vi "BonOMM-SAOMM.vi"() -> ()   [LabVIEW 2019] (continued)
                  tunnel: w3763 -> [w3827]
                  tunnel: [w3827] -> w3762
                  tunnel: w3762 -> [w3840]
                  frame #0 {
                    n5058 = Tick Count (ms)() -> (millisecond timer value=w3793:u32)
                  }
                  frame #1 {
                    # "Détecte un déplacement du télescope"
                    # "Détecte un changement de focus"
                    # "Bits du statut du TCS"
                    n5059 = Index Array(array=w3831, index #1=2 ("Index"), index #2=0 ("Index")) -> (element #1=w3812:bool, element #2=w3815:bool)
                    "Mode Est" <- w3812
                    "Focus slew" <- w3815
                    n5060 = Index Array(array=w3833, index=4 ("Index")) -> (element=w3822:bool)
                    "Target OutofRange" <- w3822
                    n5061 = Index Array(array=w3833, index=0 ("Index")) -> (element=w3804:bool)
                    n5062 = Index Array(array=w3834, index=2 ("Index")) -> (element=→"Tracking":bool)
                    n5063 = Index Array(array=w3834, index=3 ("Index")) -> (element=→"Slew enabled":bool)
                    n5064 = Index Array(array=w3834, index=4 ("indice")) -> (element=w3820:bool)
                    n5065 = Index Array(array=w3834, index=5 ("Index")) -> (element=w3821:bool)
                    "Approaching limit" <- w3821
                    n5066 = Index Array(array=w3834, index=7 ("Index")) -> (element=w3806:bool)
                    "Slewing" <- w3806
                    n5067 = Not Equal?(x=w3804, y=w3828) -> (x != y?=w3805:bool)
                    n5068 = property on="Mode Inversé" class="Bool (strict)"("Visible"=w3812, "Blinking"=w3812) -> ()  [unwired: 2 in, 2 out]
                    n5069 = property on="Target OutofRange" class="Bool (strict)"("Visible"=w3822, "Blinking"=w3822) -> ()  [unwired: 2 in, 2 out]
                    n5070 = local write "Coupole-Tél"(w3820) -> ()
                    n5071 = Not Equal?(x=w3815, y=w3829) -> (x != y?=w3814:bool)
                    n5072 = property on="Approaching limit" class="Bool (strict)"("Visible"=w3821, "Blinking"=w3821) -> ()  [unwired: 2 in, 2 out]
                    n5073 = case shown="Vrai" w3805 {
                      tunnel: w3804 -> [_ w3836]
                      frame False {
                      }
                      frame True {
                        n5074 = property on="Setting" class="Bool (strict)"("Val(Sgnl)"=w3836) -> ()  [unwired: 2 in, 2 out]
                      }
                    }
                    n5075 = case shown="Vrai" w3814 {
                      tunnel: w3815 -> [_ w3837]
                      frame False {
                      }
                      frame True {
                        n5076 = property on="Focus slew" class="Bool (strict)"("Value (Signaling)"=w3837) -> ()  [unwired: 2 in, 2 out]
                      }
                    }
                    n5077 = Not Equal?(x=w3806, y=w3830) -> (x != y?=w3807:bool)
                    n5078 = property on="Slewing" class="Bool (strict)"("Blinking"=w3806) -> ()  [unwired: 2 in, 2 out]
                    n5079 = And(x=w3804, y=w3805) -> (x .and. y?=w3808:bool)
                    n5080 = And(x=w3806, y=w3807) -> (x .and. y?=w3809:bool)
                    n5081 = local read "Servo"() -> (w3801:bool)
                    n5082 = Or(x=w3808, y=w3809) -> (x .or. y?=w3802:bool)
                    n5083 = And(x=w3802, y=w3801) -> (x .and. y?=w3803:bool)
                    n5084 = case shown="Vrai" w3803 {
                      selector: w3803 -> [_ w3835]
                      frame False {
                      }
                      frame True {
                        n5085 = property on="StopServo" class="Bool (strict)"("Val(Sgnl)"=w3835) -> ()  [unwired: 2 in, 2 out]
                      }
                    }
                    n5086 = case shown="Vrai" w3807 {
                      tunnel: w3806 -> [_ w3838]
                      frame False {
                      }
                      frame True {
                        n5087 = property on="Slewing" class="Bool (strict)"("Value (Signaling)"=w3838) -> ()  [unwired: 2 in, 2 out]
                      }
                    }
                    "STATH" <- w3833
                    "STATLH" <- w3832
                    "STATEX" <- w3831
                    "STATL" <- w3834
                  }
                  frame #2 {
                    n5088 = Tick Count (ms)() -> (millisecond timer value=w3841:u32)
                    n5089 = Subtract(x=w3841, y=w3840) -> (x-y=→"TCS #26 (sort)":u32)
                  }
                }
              }
              frame #4 {
                n5090 = Tick Count (ms)() -> (millisecond timer value=w3844:u32)
                n5091 = Subtract(x=w3844, y=w3843) -> (x-y=→"TCS #26":u32)
              }
              frame #5 {
                # "Malheureusement, semble causé un problème \nquand on tente de reconnecté les tables ...\nChecher à comprendre c'Est avoir mal à la tête\nprobablement un VI non-réentrant partager entre\nle query de TCS et le query des tables ..."
                # "Patch pour l'angle (2013/06/22)\nÀ mettre au propre ... attention,\ncela à beaucoup d'impact sur beaucou\nde sous-routine ... (voir tout ce qui re-\nçoit l'angle à un moment)"
                # "À remettre dans un mode correct"
                n5092 = local read "TCSMute"() -> (w3845:bool)
                n5093 = local read "TCS VRN"() -> (w3858:refnum<visa-resource-name>)
                n5094 = control-ref of="TCS actif"() -> (w3856:refnum<vi>)
                n5095 = local read "dflt-EQX"() -> (w3855:dbl)
                n5096 = case shown="Faux" w3845 {
                  tunnel: [w3896 w3897] -> w3879
                  tunnel: [w3895 w3897] -> w3878
                  tunnel: [w3894 w3897] -> w3877
                  tunnel: [w3893 w3897] -> w3876
                  tunnel: [w3892 ""] -> w3875
                  tunnel: [w3891 w3897] -> w3868
                  tunnel: [w3890 w3897] -> w3867
                  tunnel: [w3889 w3897] -> w3866
                  tunnel: [w3888 w3897] -> w3865
                  tunnel: [w3887 errorcluster {"status"=FALSE, "code"=0, "source"=""} ("Error OUT")] -> w3864
                  tunnel: [w3886 w3900] -> w3859
                  tunnel: w3858 -> [w3885 w3900]
                  tunnel: w3856 -> [w3884 _]
                  tunnel: w3855 -> [w3883 _]
                  tunnel: [w3882 w3897] -> w3853
                  tunnel: [w3881 w3897] -> w3852
                  tunnel: [w3880 w3897] -> w3848
                  frame False {
                    n5097 = call "EXCOM-25-EQ.vi"("VISA resource name"=w3885, "Bool Refnum"=w3884, "Display Equinox"=w3883) -> ("HA"=w3893:dbl, "Q String"=w3892:string, "RA"=w3881:dbl, "Rotateur"=w3880:dbl, "DEC"=w3882:dbl, "Dome"=w3896:dbl, "Epoque"=w3891:dbl, "Focus"=w3895:dbl, "VISA resource name dup"=w3886:refnum<visa-resource-name>, "Masse d'air"=w3894:dbl, "Temps Sidéral"=w3890:dbl, "Temps Universel"=w3889:dbl, "Année"=w3888:dbl, "Error OUT"=w3887:errorcluster)  [unwired: 2 in, 1 out]
                  }
                  frame True {
                    w3897 = 0.0
                  }
                }
                "Q String" <- w3875
                "RA Tel" <- w3852
                "DEC Tel" <- w3853
                "Angle Hor." <- w3876
                "Epoch Tel" <- w3868
                "Air Mass" <- w3877
                "LST" <- w3867
                "UTC" <- w3866
                "AnnéeRL" <- w3865
                "Foyer" <- w3878
                "Coupole" <- w3879
                n5098 = call-poly "PolyCommError.vi"("VISA IN"=w3859, "error IN"=w3864) -> ("VISA OUT"=w3857:refnum<visa-resource-name>, "Error"=w3860:bool)  [unwired: 11 in, 1 out]
                n5099 = Not(x=w3860) -> (.not. x?=w3854:bool)
                n5100 = local write "Sync_Ready"(w3854) -> ()
                n5101 = Add(x=w3848, y="Ajustement fin de rotation") -> (x+y=w3847:dbl)
                "RotationTCS" <- w3847
                n5102 = local write "TCS VRN"(w3857) -> ()
                n5103 = Negate(x=w3847) -> (-x=w3851:dbl)
                n5104 = local read "N.O. Déc."() -> (w3870:string)
                n5105 = local read "N.O. A.D."() -> (w3872:string)
                n5106 = Add(x=w3851, y=90.0) -> (x+y=→"RotationEffective":dbl)
                n5107 = local read "NO epoch"() -> (w3869:dbl)
                n5108 = call "time-str-to-time-dbl-RA.vi"("Chaîne"=w3872) -> ("TCS_coords"=w3871:dbl)
                n5109 = call "time-str-to-time-dbl-DEC.vi"("Chaîne"=w3870) -> ("TCS_coords"=w3862:dbl)
                n5110 = expression code="x*3600"(w3871) -> (w3863:dbl)
                n5111 = expression code="x*3600"(w3862) -> (w3861:dbl)
                n5112 = call "Object_properties.vi"("Target RA"=w3863, "Target DEC"=w3861, "Target Epoch"=w3869, "Sideral Time"=w3867) -> ("NO HA"=w3874:dbl, "NO AM"=w3873:dbl)  [unwired: 7 in, 3 out]
                n5113 = local write "NO AM"(w3873) -> ()
                n5114 = local write "NO HA"(w3874) -> ()
              }
              frame #6 {
                n5115 = Tick Count (ms)() -> (millisecond timer value=w3902:u32)
                n5116 = Subtract(x=w3902, y=w3903) -> (x-y=→"TCS #25":u32)
              }
              frame #7 {
                n5117 = local read "Position X"() -> (w3906:dbl)
                n5118 = local read "Position Z"() -> (w3904:dbl)
                n5119 = local read "Position Y"() -> (w3905:dbl)
              }
              frame #8 {
                n5120 = Tick Count (ms)() -> (millisecond timer value=w3911:u32)
                n5121 = local read "TableMute"() -> (w3907:bool)
                n5122 = case shown="Faux" w3907 {
                  tunnel: w3910 -> [w3919 _]
                  tunnel: w3909 -> [w3918 _]
                  tunnel: w3908 -> [w3917 _]
                  frame False {
                    # "Si on tente une reconnexion, on empêche le query ..."
                    n5123 = local read "Table Error"() -> (w3927:errorcluster)
                    n5124 = local read "Table VRN"() -> (w3928:refnum<visa-resource-name>)
                    n5125 = control-ref of="Table actif"() -> (w3929:refnum<vi>)
                    n5126 = call "Newmark-QueryPosition.vi"("Table VRN IN"=w3928, "Bool Refnum"=w3929, "Error IN"=w3927) -> ("X Axis"=w3923:dbl, "Y Axis"=w3922:dbl, "Table VRN OUT"=w3926:refnum<visa-resource-name>, "Exception"=w3924:string, "Z Axis"=w3916:dbl, "Error OUT"=w3925:errorcluster)  [unwired: 5 in, 2 out]
                    "Position X" <- w3923
                    "Position Y" <- w3922
                    "Position Z" <- w3916
                    n5127 = flat-sequence {
                      tunnel: w3924 -> [w3936]
                      tunnel: [w3936] -> w3932
                      tunnel: w3932 -> [w3939]
                      frame #0 {
                        n5128 = control-ref of="Table actif"() -> (w3938:refnum<vi>)
                        n5129 = call "Newmark-Wait4Flag.vi"("Raise Flag ?"=TRUE, "Ctl Refnum IN"=w3938) -> ()  [unwired: 8 in, 2 out]
                      }
                      frame #1 {
                        n5130 = local read "Exceptions"() -> (w3941:T3)
                        n5131 = call "ExceptionStacker.vi"("ExceptionString"=w3939, "Newmark-Exceptions IN"=w3941) -> ("Newmark-Exceptions OUT"=w3940:T3)  [unwired: 13 in]
                        n5132 = local write "Exceptions"(w3940) -> ()
                      }
                      frame #2 {
                        n5133 = local write "Table actif"(FALSE ("Table actif")) -> ()
                      }
                    }
                    n5134 = Not Equal?(x=w3919, y=w3923) -> (x != y?=w3921:bool)
                    n5135 = Not Equal?(x=w3918, y=w3922) -> (x != y?=w3920:bool)
                    n5136 = local write "Table Error"(w3925) -> ()
                    n5137 = Or(x=w3921, y=w3920) -> (x .or. y?=w3912:bool)
                    n5138 = local write "Table VRN"(w3926) -> ()
                    n5139 = local write "MovingXY"(w3912) -> ()
                    n5140 = local write "Indicateur d'état"("Lecture des paramètres des tables" ("Indicateur d'état")) -> ()
                    n5141 = local write "FoyerTable"(w3916) -> ()
                    n5142 = Not Equal?(x=w3916, y=w3917) -> (x != y?=w3915:bool)
                    n5143 = local write "MovingZ"(w3915) -> ()
                    n5144 = local read "Origine en cours..."() -> (w3913:bool)
                    n5145 = Or(x=w3912, y=w3913) -> (x .or. y?=w3914:bool)
                    n5146 = case shown="Vrai" w3914 {
                      frame False {
                        # "Désactive les boutons quand la position \ncible est différente de la position lue."
                        n5147 = local read "CorrectXY"() -> (w3933:bool)
                        n5148 = case shown="Faux" w3933 {
                          frame False {
                            w3934 = T17."Enabled" ("Disabled")
                            n5149 = property on="Centre" class="Bool (strict)"("Disabled"=w3934) -> ()  [unwired: 2 in, 2 out]
                            n5150 = property on="Alacible" class="Bool (strict)"("Disabled"=w3934) -> ()  [unwired: 2 in, 2 out]
                            n5151 = property on="Origine" class="Bool (strict)"("Disabled"=w3934) -> ()  [unwired: 2 in, 2 out]
                            n5152 = property on="go Est" class="Bool (strict)"("Disabled"=w3934) -> ()  [unwired: 2 in, 2 out]
                            n5153 = property on="Calibration" class="Bool (strict)"("Disabled"=w3934) -> ()  [unwired: 2 in, 2 out]
                            n5154 = property on="Centrage" class="Bool"("Disabled"=w3934) -> ()  [unwired: 2 in, 2 out]
                            n5155 = property on="go Sud" class="Bool (strict)"("Disabled"=w3934) -> ()  [unwired: 2 in, 2 out]
                            n5156 = property on="RangeTable" class="Bool (strict)"("Disabled"=w3934) -> ()  [unwired: 2 in, 2 out]
                            n5157 = property on="Foyer+" class="Bool (strict)"("DisabledEnum"=w3934) -> ()  [unwired: 2 in, 2 out]
                            n5158 = property on="go Ouest" class="Bool (strict)"("Disabled"=w3934) -> ()  [unwired: 2 in, 2 out]
                            n5159 = property on="Foyer-" class="Bool (strict)"("DisabledEnum"=w3934) -> ()  [unwired: 2 in, 2 out]
                            n5160 = property on="go Nord" class="Bool (strict)"("Disabled"=w3934) -> ()  [unwired: 2 in, 2 out]
                          }
                          frame True {
                          }
                        }
                      }
                      frame True {
                        w3935 = T17."Disabled and Grayed Out" ("Disabled")
                        n5161 = property on="Centre" class="Bool (strict)"("Disabled"=w3935) -> ()  [unwired: 2 in, 2 out]
                        n5162 = property on="Alacible" class="Bool (strict)"("Disabled"=w3935) -> ()  [unwired: 2 in, 2 out]
                        n5163 = property on="Origine" class="Bool (strict)"("Disabled"=w3935) -> ()  [unwired: 2 in, 2 out]
                        n5164 = property on="go Est" class="Bool (strict)"("Disabled"=w3935) -> ()  [unwired: 2 in, 2 out]
                        n5165 = property on="Calibration" class="Bool (strict)"("Disabled"=w3935) -> ()  [unwired: 2 in, 2 out]
                        n5166 = property on="Centrage" class="Bool"("Disabled"=w3935) -> ()  [unwired: 2 in, 2 out]
                        n5167 = property on="go Sud" class="Bool (strict)"("Disabled"=w3935) -> ()  [unwired: 2 in, 2 out]
                        n5168 = property on="RangeTable" class="Bool (strict)"("Disabled"=w3935) -> ()  [unwired: 2 in, 2 out]
                        n5169 = property on="Foyer+" class="Bool (strict)"("DisabledEnum"=w3935) -> ()  [unwired: 2 in, 2 out]
                        n5170 = property on="go Ouest" class="Bool (strict)"("Disabled"=w3935) -> ()  [unwired: 2 in, 2 out]
                        n5171 = property on="Foyer-" class="Bool (strict)"("DisabledEnum"=w3935) -> ()  [unwired: 2 in, 2 out]
                        n5172 = property on="go Nord" class="Bool (strict)"("Disabled"=w3935) -> ()  [unwired: 2 in, 2 out]
                      }
                    }
                    "TabQstr" <- ""
                  }
                  frame True {
                  }
                }
              }
              frame #9 {
                # "Détecte un arrêt du stage Z"
                # "Détecte un arrêt des tables XY\nMovingXY -> était vrai, devient faux"
                # "Détection de l'arrêt des tables de translation ..."
                n5173 = local read "MovingZ"() -> (w3944:bool)
                n5174 = local read "MovingXY"() -> (w3949:bool)
                n5175 = Not(x=w3944) -> (.not. x?=w3945:bool)
                n5176 = And(x=w3946, y=w3945) -> (x .and. y?=w3943:bool)
                n5177 = Not(x=w3949) -> (.not. x?=w3948:bool)
                n5178 = And(x=w3950, y=w3948) -> (x .and. y?=w3947:bool)
                n5179 = case shown="Vrai" w3947 {
                  frame False {
                  }
                  frame True {
                    # "Détecte un arrêt des étages XY"
                    n5180 = flat-sequence {
                      frame #0 {
                        n5181 = local read "CorrectXY"() -> (w3971:bool)
                        n5182 = case shown="Vrai" w3971 {
                          frame False {
                          }
                          frame True {
                            n5183 = local write "CorrectXY"(FALSE ("CorrectXY")) -> ()
                            n5184 = property on="ApplyCorrection" class="Bool (strict)"("Val(Sgnl)"=TRUE ("Value (Signaling)")) -> ()  [unwired: 2 in, 2 out]
                          }
                        }
                      }
                      frame #1 {
                        n5185 = local read "CurvCorrect"() -> (w3974:bool)
                        n5186 = case shown="Vrai" w3974 {
                          frame False {
                          }
                          frame True {
                            n5187 = local read "CentreTel X"() -> (w3984:dbl)
                            n5188 = local read "CentreTel Y"() -> (w3983:dbl)
                            n5189 = local read "Position X"() -> (w3977:dbl)
                            n5190 = local read "Position Y"() -> (w3976:dbl)
                            n5191 = local read "FoyerAuCentre"() -> (w3980:dbl)
                            n5192 = call "Calc_focus.vi"("Pos X"=w3977, "a0"=w3980, "Pos Y"=w3976, "Cen X"=w3984, "Cen Y"=w3983, "a1"="a1_focus", "a2"="a2_focus", "a3"="a3_focus") -> ("Foyer"=w3982:dbl)  [unwired: 6 in, 1 out]
                            n5193 = local write "CurvCorrect"(FALSE ("CorrectZ")) -> ()
                            n5194 = property on="FoyerTable" class="NumNb (strict)"("Val(Sgnl)"=w3982) -> ()  [unwired: 2 in, 2 out]
                          }
                        }
                      }
                    }
                  }
                }
                n5195 = case shown="Vrai" w3943 {
                  frame False {
                  }
                  frame True {
                    # "Détecte un arrêt de l'étage de foyer"
                    n5196 = flat-sequence {
                      tunnel: [w3952] -> w3951
                      tunnel: w3951 -> [w3959]
                      frame #0 {
                        n5197 = local read "CorrectZ"() -> (w3953:bool)
                        n5198 = case shown="Vrai" w3953 {
                          tunnel: [w3954 w3955] -> w3952
                          frame False {
                            n5199 = local read "Position Z"() -> (w3954:dbl)
                          }
                          frame True {
                            n5200 = local read "Cible Z"() -> (w3955:dbl)
                            n5201 = local write "CorrectZ"(FALSE ("CorrectZ")) -> ()
                            n5202 = property on="ApplyCorrection" class="Bool (strict)"("Val(Sgnl)"=TRUE ("Value (Signaling)")) -> ()  [unwired: 2 in, 2 out]
                          }
                        }
                      }
                      frame #1 {
                        # "Ajuste le foyer en fonction du nombre de pas à partir du centre"
                        n5203 = local read "Focusing"() -> (w3958:bool)
                        n5204 = case shown="Vrai" w3958 {
                          tunnel: w3959 -> [_ w3961]
                          frame False {
                          }
                          frame True {
                            n5205 = local read "Reference X"() -> (w3967:dbl)
                            n5206 = local read "Reference Y"() -> (w3968:dbl)
                            n5207 = local read "Position X"() -> (w3962:dbl)
                            n5208 = local read "Position Y"() -> (w3963:dbl)
                            n5209 = local read "a1_focus"() -> (w3969:dbl)
                            n5210 = local read "a2_focus"() -> (w3965:dbl)
                            n5211 = local read "a3_focus"() -> (w3966:dbl)
                            n5212 = call "Calc_focus.vi"("Pos X"=w3962, "Pos Y"=w3963, "Cen X"=w3967, "Cen Y"=w3968, "a1"=w3969, "a2"=w3965, "a3"=w3966) -> ("Residu"=w3964:dbl)  [unwired: 7 in, 1 out]
                            n5213 = Subtract(x=w3961, y=w3964) -> (x-y=w3970:dbl)
                            n5214 = local write "Focusing"(FALSE ("Focusing")) -> ()
                            n5215 = local write "FoyerAuCentre"(w3970) -> ()
                          }
                        }
                      }
                    }
                  }
                }
              }
              frame #10 {
                w4055 = u16 0 items=["Square", "Circle"] ("Ring")
                # "Calcul des astrométries et positions ..."
                # "Invert X"
                # "Redessine la représentation du champ"
                # "Réinitialise le data USNO"
                # "Réinitialise l'image"
                # "Vérifie si les données sont encore actuelles ..."
                # "Nombre d'arcsec\nd'écart acceptées"
                # "Époque DSS et USNO"
                # "Calcul la position de la sonde ..."
                # "Refait avec les nouvelles astrométries ..."
                n5216 = Tick Count (ms)() -> (millisecond timer value=w4067:u32)
                n5217 = Subtract(x=w4067, y=w4068) -> (x-y=→"Table Q":u32)
                n5218 = local read "Binning"() -> (w4003:u16)
                n5219 = local read "Dec Sonde"() -> (w3999:dbl)
                n5220 = local read "PixScale1"() -> (w4005:dbl)
                n5221 = local read "PixScale2"() -> (w4004:dbl)
                n5222 = local read "RA Sonde"() -> (w4000:dbl)
                n5223 = local read "Naxis1"() -> (w4006:u16)
                n5224 = local read "Naxis2"() -> (w4007:u16)
                n5225 = local read "RotationEffective"() -> (w3997:dbl)
                n5226 = local read "Reference Y"() -> (w4013:dbl)
                n5227 = local read "Reference X"() -> (w4014:dbl)
                n5228 = local read "RotationEffective"() -> (w3996:dbl)
                n5229 = local read "CentreTel X"() -> (w4016:dbl)
                n5230 = local read "CentreTel Y"() -> (w4015:dbl)
                n5231 = Bundle("Naxis1"=w4006, "Naxis2"=w4007) -> (w4001:cluster{"Naxis1":u16, "Naxis2":u16})  [unwired: 1 in]
                n5232 = Bundle("PixScale1"=w4005, "PixScale2"=w4004) -> (w4002:cluster{"PixScale1":dbl, "PixScale2":dbl})  [unwired: 1 in]
                n5233 = local read "arcsec/pulse"() -> (w4057:dbl)
                n5234 = call "SAOMM-Astrometry.vi"("Binning"=w4003, "PIXSCALE"=w4002, "NAXIS"=w4001, "Rotation"=w3997, "RAsonde"=w4000, "DECsonde"=w3999) -> ("GuideAstrom"=w3998:T4)  [unwired: 9 in]
                n5235 = local read "DEC Tel"() -> (w4060:dbl)
                n5236 = local read "RA Tel"() -> (w4061:dbl)
                n5237 = local write "GuiderAstrom"(w3998) -> ()
                n5238 = local read "Représentation"() -> (w4029:dbl)
                n5239 = property on="TableXYPos" class="GraphXY (strict)"("Active Cursor"=u32 1) -> ("Cursor.Cursor X"=w3991:dbl, "Cursor.Cursor Y"=w3990:dbl)  [unwired: 2 in, 2 out]
                n5240 = local read "MirVig"() -> (w3993:dbl)
                n5241 = local read "MirFOV"() -> (w3988:dbl)
                n5242 = local read "Miroir"() -> (w3992:dbl)
                n5243 = call "Set_field_astrometry.vi"("Cen x (pas)"=w4016, "effective rotation (°)"=w3996, "scale (\"/pas)"=w4057, "NaxisMax"=500000, "Cen y (pas)"=w4015, "Use Center?"=FALSE ("Ues Constant Size ?"), "Ref x (pas)"=w4014, "Ref y (pas)"=w4013, "RA (HH:MM:SS.S)"=w4061, "DEC(DD:MM:SS)"=w4060, "Inversion Cluster"=T20 {"Invert Angle"=FALSE, "Invert X"=TRUE, "Invert Y"=FALSE}) -> ("Field Astrometry"=w4053:T4, "Table Astrometry"=w4054:T4)  [unwired: 3 in]
                n5244 = local read "BrasPesto"() -> (w3985:bool)
                n5245 = local read "LimXPesto"() -> (w3986:dbl)
                n5246 = local read "FOV"() -> (w4056:dbl)
                n5247 = Bundle("Miroir"=w3992, "Cursor.Cursor X"=w3991, "Cursor.Cursor Y"=w3990, "MirVig"=w3993, "MirFOV"=w3988, "LimXPesto"=w3986, "BrasPesto"=w3985) -> (w3989:T48)  [unwired: 1 in]
                n5248 = local read "NaxisMax"() -> (w4012:dbl)
                n5249 = local read "RotationEffective"() -> (w3987:dbl)
                n5250 = call "draw_field.vi"("Field_Astrometry"=w4053, "FOV"=w4056, "NaxisMax"=w4012, "Ring"=w4055, "Table_Astrometry"=w4054, "Rotation effective"=w3987, "Ues Constant Size ?"=TRUE, "margin/size"=w4029, "MirrorAvatar"=w3989) -> ("TableXYPos"=w4039:cluster{dbl[], dbl[]}[], "X Scale.Range"=w4040:T26, "ImgDEC"=w3995:dbl, "ImgRA"=w4050:dbl, "Y Scale.Range"=w4038:T26)  [unwired: 2 in]
                n5251 = local read "Epoch Tel"() -> (w4051:dbl)
                n5252 = local read "DEC-USNO"() -> (w4023:dbl)
                n5253 = local write "FieldAstrom"(w4053) -> ()
                n5254 = local write "TableAstrom"(w4054) -> ()
                n5255 = local read "RA-USNO"() -> (w4024:dbl)
                n5256 = local read "Position X"() -> (w4010:dbl)
                n5257 = local read "Position Y"() -> (w4009:dbl)
                n5258 = call "precess.vi"("Eq2"=2000.0, "Eq1"=w4051, "DEC 1"=w3995, "RA 1"=w4050) -> ("DEC 2"=w4027:dbl, "RA 2"=w4028:dbl)
                "RA-Champ" <- w4028
                "DEC-Champ" <- w4027
                n5259 = call "xy2ad.vi"("Y (px)"=w4009, "X (px)"=w4010, "Astrometry"=w4054) -> ("DEC (°)"=w4062:dbl, "RA (°)"=w4063:dbl, "DEC (HH:MM:SS)"=→"Dec Sonde":dbl, "RA (HH:MM:SS.S)"=→"RA Sonde":dbl)  [unwired: 5 in]
                n5260 = local read "Img DEC"() -> (w4017:dbl)
                n5261 = local read "Img RA"() -> (w4018:dbl)
                n5262 = call "deg2ad.vi"("DEC (°)"=w4027, "RA (°)"=w4028) -> ("DEC (°)"=→"DEC-Champ-sec":dbl, "RA (sec)"=→"RA-Champ-sec":dbl)
                n5263 = call "deg2ad.vi"("DEC (°)"=w4023, "RA (°)"=w4024) -> ("DEC (°)"=→"DEC-USNO-sec":dbl, "RA (sec)"=→"RA-USNO-sec":dbl)
                n5264 = flat-sequence {
                  tunnel: w4063 -> [w4093]
                  tunnel: w4062 -> [w4092]
                  tunnel: w4053 -> [w4091]
                  tunnel: [w4090] -> w4041
                  tunnel: w4040 -> [w4088]
                  tunnel: w4039 -> [w4087]
                  tunnel: w4038 -> [w4086]
                  tunnel: w4041 -> [w4095]
                  frame #0 {
                    # "Calcul la position de la cible"
                    n5265 = call "ad2xy.vi"("DEC"=w4092, "RA"=w4093, "Astrometry"=w4091) -> ("Y"=w4084:dbl, "X"=w4085:dbl, "Dup Astrometry"=w4090:T4)  [unwired: 6 in]
                    n5266 = call "format_arcmin2arcsecstr.vi"("RA arcmin"=w4085, "DEC Arcmin"=w4084) -> ("Formatted RA"=→"Cen-Snd-RA":string, "Formatted Dist"=→"Cen-Snd-TOT":string, "Formatted DEC"=→"Cen-Snd-DEC":string)  [unwired: 11 in]
                    n5267 = property on="TableXYPos" class="GraphXY (strict)"("Active Cursor"=u32 1, "Cursor.Cursor X"=w4085, "Cursor.Cursor Y"=w4084, "Value"=w4087, "XScale.Range"=w4088, "YScale.Range"=w4086) -> ()  [unwired: 2 in, 2 out]
                  }
                  frame #1 {
                    n5268 = case shown="Faux" "CursorLock" {
                      tunnel: w4095 -> [w4101 _]
                      frame False {
                        n5269 = property on="TableXYPos" class="GraphXY (strict)"("Active Cursor"=u32 0) -> ("Cursor.Cursor X"=w4100:dbl, "Cursor.Cursor Y"=w4099:dbl)  [unwired: 2 in, 2 out]
                        n5270 = call "format_arcmin2arcsecstr.vi"("RA arcmin"=w4100, "DEC Arcmin"=w4099) -> ("Formatted RA"=w4096:string, "Formatted Dist"=→"Cen-Cib-TOT":string, "Formatted DEC"=w4097:string)  [unwired: 11 in]
                        n5271 = call "xy2ad.vi"("Y (px)"=w4099, "X (px)"=w4100, "Astrometry"=w4101) -> ("DEC (HH:MM:SS)"=→"Dec Cible":dbl, "RA (HH:MM:SS.S)"=→"RA Cible":dbl)  [unwired: 5 in, 2 out]
                        n5272 = local write "Cen-Cib-RA"(w4096) -> ()
                        n5273 = local write "Cen-Cib-DEC"(w4097) -> ()
                      }
                      frame True {
                      }
                    }
                  }
                }
                n5274 = expression code="x/3600"(5.0) -> (w4031:dbl)
                n5275 = call "deg2ad.vi"("DEC (°)"=w4017, "RA (°)"=w4018) -> ("DEC (°)"=→"DEC-DSS-sec":dbl, "RA (sec)"=→"RA-DSS-sec":dbl)
                n5276 = Subtract(x=w4028, y=w4018) -> (x-y=w4049:dbl)
                n5277 = Subtract(x=w4028, y=w4024) -> (x-y=w4032:dbl)
                n5278 = Subtract(x=w4027, y=w4017) -> (x-y=w4048:dbl)
                n5279 = Subtract(x=w4027, y=w4023) -> (x-y=w4033:dbl)
                n5280 = Absolute Value(x=w4048) -> (abs(x)=w4045:dbl)
                n5281 = Absolute Value(x=w4033) -> (abs(x)=w4035:dbl)
                n5282 = Absolute Value(x=w4049) -> (abs(x)=w4047:dbl)
                n5283 = Absolute Value(x=w4032) -> (abs(x)=w4034:dbl)
                n5284 = Greater?(x=w4047, y=w4031) -> (0:w4044:bool)
                n5285 = Greater?(x=w4045, y=w4031) -> (0:w4043:bool)
                n5286 = Greater?(x=w4034, y=w4031) -> (0:w4036:bool)
                n5287 = Greater?(x=w4035, y=w4031) -> (0:w4037:bool)
                n5288 = Or(x=w4044, y=w4043) -> (x .or. y?=w4042:bool)
                n5289 = Or(x=w4036, y=w4037) -> (x .or. y?=w4030:bool)
                n5290 = case shown="Vrai" w4030 {
                  frame False {
                  }
                  frame True {
                    w4074 = 0
                    n5291 = local read "SubIMG4DSS?"() -> (w4070:bool)
                    n5292 = local read "Integrating"() -> (w4072:bool)
                    n5293 = Initialize Array(sgl 0.0, w4074, w4074) -> (w4073:sgl[][])
                    n5294 = local write "BestTargetLed"(FALSE) -> ()
                    n5295 = local write "ImgData"(w4073) -> ()
                    n5296 = Not(x=w4072) -> (.not. x?=w4071:bool)
                    n5297 = And(x=w4070, y=w4071) -> (x .and. y?=w4069:bool)
                    n5298 = case shown="Vrai" w4069 {
                      tunnel: w4073 -> [_ w4080]
                      frame False {
                      }
                      frame True {
                        w4077 = u16 2 items=["Region d'intérêt", "Prévisualisation", "Idle"] ("ImageUsage")
                        n5299 = call "Draw_crosshair.vi"("Image IN"=w4080, "White Value"=sgl 255.0) -> ("Image OUT"=w4079:sgl[][])  [unwired: 13 in]
                        n5300 = local write "ImageUsage"(w4077) -> ()
                        n5301 = local write "subimg"(w4079) -> ()
                      }
                    }
                  }
                }
                n5302 = case shown="Vrai" w4042 {
                  frame False {
                  }
                  frame True {
                    w4105 = FALSE ("ImageDSSLed")
                    n5303 = local write "ImageDSSLed"(w4105) -> ()
                    n5304 = property on="TableXYPos" class="GraphXY (strict)"("PlotImages.Back"=picture data[5B] ("Plot Images:Back")) -> ()  [unwired: 2 in, 2 out]
                    n5305 = local write "DS9-Led"(w4105) -> ()
                  }
                }
              }
              frame #11 {
                # "Ajout des données des LVDTs"
                n5306 = Tick Count (ms)() -> (millisecond timer value=w4109:u32)
                n5307 = Subtract(x=w4109, y=w4111) -> (x-y=→"TotalExecTime":u32)
                n5308 = Subtract(x=w4109, y=w4108) -> (x-y=→"CursorSet":u32)
              }
              frame #12 {
                # "Boucle des Alarmes sonores"
                n5309 = stacked-sequence {
                  frame #0 {
                    w4119 = 3600
                    # "Dec min pour collision"
                    # "Limite  angle horaire B"
                    # "Limite  angle horaire A"
                    # "CPAPIR proche du pillier"
                    n5310 = local read "AS_B_Pillier"() -> (w4113:bool)
                    n5311 = local read "DEC Tel"() -> (w4120:dbl)
                    n5312 = local read "Angle Hor."() -> (w4124:dbl)
                    n5313 = Multiply(x=3.0 ("y"), y=w4119) -> (x*y=w4123:dbl)
                    n5314 = Multiply(x=w4119, y=60.0) -> (x*y=w4117:dbl)
                    n5315 = Multiply(x=7.0 ("y"), y=w4119) -> (x*y=w4126:dbl)
                    n5316 = Greater?(x=w4126, y=w4124) -> (0:w4122:bool)
                    n5317 = Greater?(x=w4124, y=w4123) -> (0:w4121:bool)
                    n5318 = Greater?(x=w4120, y=w4117) -> (0:w4115:bool)
                    n5319 = And(x=w4122, y=w4121) -> (x .and. y?=w4116:bool)
                    n5320 = And(x=w4116, y=w4115) -> (x .and. y?=w4114:bool)
                    n5321 = And(x=w4114, y=w4113) -> (x .and. y?=w4112:bool)
                    n5322 = local write "AS_I_Pillier"(w4112) -> ()
                  }
                }
              }
            }
            n5323 = Wait Until Next ms Multiple(millisecond multiple=u32 200) -> ()  [unwired: 1 out]
            n5324 = local read "Quit"() -> (w3648:bool)
            n5325 = Tick Count (ms)() -> (millisecond timer value=w3663:u32)
          }
          "Query et Status" <- w979
          n5326 = while {
            tunnel: [w3405] -> w978
            i -> [w3406]
            stop <- w3405 stop-if-true
            # "À passer dans une boucle périodique à plusieurs étages parce que c'est le bordel."
            # "Structure de gestion des événements software"
            n5327 = event shown="[2] \"Recalculer\": Valeur changée" {
              selector: _ -> [_ _ _ _]
              dyn-events: _ -> [_ _ _ _]
              timeout: 250 -> [_ _ _ _]
              tunnel: w3406 -> [w3409 _ _ _]
              event Timeout {
                # "Au ~30 sec ..."
                # "Reconnection/Acquisition des donneés météo ..."
                # "Au ~10 secondes ..."
                n5328 = event-data() -> ()  [unwired: 1 in, 2 out]
                n5329 = Quotient & Remainder(x=w3409, y=40) -> (x-y*floor(x/y)=w3413:i32)  [unwired: 1 out]
                n5330 = Equal To 0?(x=w3413) -> (x = 0?=w3412:bool)
                n5331 = case shown="Vrai" w3412 {
                  frame False {
                  }
                  frame True {
                    n5332 = stacked-sequence {
                      frame #0 {
                        # "Si le foyer reste constant pendant plus de 5 minutes, on suppose que le foyer a été fait et est correct ..."
                        n5333 = local read "CheckFocus"() -> (w3421:bool)
                        n5334 = case shown="Vrai" w3421 {
                          frame False {
                          }
                          frame True {
                            n5335 = local read "last_foc_chg"() -> (w3425:ext)
                            n5336 = Get Date/Time In Seconds() -> (seconds since 1Jan1904=w3427:timestamp)
                            n5337 = To Extended Precision Float(1:w3427) -> (0:w3426:ext)
                            n5338 = Subtract(x=w3426, y=w3425) -> (x-y=w3424:ext)
                            n5339 = Greater?(x=w3424, y=ext 300.0) -> (0:w3422:bool)
                            n5340 = case shown="Vrai" w3422 {
                              frame False {
                              }
                              frame True {
                                # "Si il y a une connexion à\nla station météo ..."
                                # "Une fois que le comportement aura été testé, on pourra\nécrire le résultat dans le fichier \"instruments.ini\""
                                n5341 = local read "Cx"() -> (w3429:bool)
                                n5342 = case shown="Vrai" w3429 {
                                frame False {
                                }
                                frame True {
                                # "On enregistre les données ..."
                                n5343 = local read "indic-T-out"() -> (w3431:dbl)
                                n5344 = local read "indic-T-in"() -> (w3430:dbl)
                                n5345 = local read "path_focuslog"() -> (w3432:path)
                                n5346 = local read "Instrument Actuel"() -> (w3433:string)
                                n5347 = local read "tmp.str"() -> (w3434:dbl)
                                n5348 = local read "Foyer Nominal"() -> (w3435:dbl)
                                n5349 = call "write_focus_file.vi"("Log_dir"=w3432, "Instrument"=w3433, "Foyer"=w3435, "Temp.str"=w3434, "Temp.int"=w3430, "Temp.ext"=w3431) -> ()  [unwired: 6 in]
                                n5350 = local read "Ath_coef"() -> (w3439:dbl)
                                n5351 = Multiply(x=w3439, y=w3434) -> (x*y=w3438:dbl)
                                n5352 = Subtract(x=w3435, y=w3438) -> (x-y=w3437:dbl)
                                n5353 = To Long Integer(number=w3437) -> (32bit integer=w3436:i32)
                                n5354 = local write "Foyer à 0°"(w3436) -> ()
                                }
                                }
                                n5355 = local write "CheckFocus"(FALSE ("CheckFocus")) -> ()
                              }
                            }
                          }
                        }
                      }
                      frame #1 {
                        # "Modification du foyer par une \ndifférence de température ..."
                        # "Éventuellement à calculer à partir\ndes données instrumentales ..."
                        n5356 = local read "indic-T-struct"() -> (w3445:dbl)
                        n5357 = local read "tmp.str"() -> (w3440:dbl)
                        n5358 = local read "Bypass Auto-focus"() -> (w3446:bool)
                        n5359 = Subtract(x=w3440, y=w3445) -> (x-y=w3444:dbl)
                        n5360 = Absolute Value(x=w3444) -> (abs(x)=w3443:dbl)
                        n5361 = Greater?(x=w3443, y=2.0) -> (0:w3441:bool)
                        n5362 = And(x=w3446, y=w3441) -> (x .and. y?=w3447:bool)
                        n5363 = case shown="Vrai" w3447 {
                          tunnel: w3440 -> [_ w3452]
                          frame False {
                          }
                          frame True {
                            n5364 = local read "Foyer à 0°"() -> (w3451:i32)
                            n5365 = local read "Ath_coef"() -> (w3449:dbl)
                            n5366 = To Double Precision Float(number=w3451) -> (double precision float=w3450:dbl)
                            n5367 = call "Athermalize-focus.vi"("Coefficient Thermique"=w3449, "temperature actuelle"=w3452, "Foyer à 0°"=w3450) -> ("Foyer suggérer"=w3448:i32)  [unwired: 1 in]
                            n5368 = Number To Decimal String(number=w3448) -> (decimal integer string=w3461:string)  [unwired: 1 in]
                            n5369 = Concatenate Strings("La température a suffisamment changée\npour justifier un ajustement du foyer ...\nDésirez-vous faire l'ajustement maintenant ?\n(Valeur suggérée : " ("message"), w3461, " ADU)" ("string")) -> (w3459:string)
                            n5370 = call <vilib>:"Three Button Dialog.vi"("Allow user to close window? (TRUE)"=FALSE, "Justify Message (Left)"=enum16{"Left", "Center", "Right"}."Center", "Right Button Text (\"Cancel\")"="Ne plus me demander" ("string"), "Center Button Text (\"No\")"="NON" ("string"), "Left Button Text (\"Yes\")"="OUI" ("string"), "message"=w3459) -> ("Which Button?"=w3458:T61)  [unwired: 5 in]
                            n5371 = case shown="\"Center Button\"" w3458 {
                              frame "Left Button", Default {
                              }
                              frame "Center Button" {
                                n5372 = local read "indic-T-struct"() -> (w3463:dbl)
                                n5373 = local write "tmp.str"(w3463) -> ()
                              }
                              frame "Right Button" {
                                "Bypass Auto-focus" <- TRUE ("Allow user to close window? (TRUE)")
                              }
                            }
                          }
                        }
                      }
                    }
                  }
                }
                n5374 = Quotient & Remainder(x=w3409, y=10) -> (x-y*floor(x/y)=w3411:i32)  [unwired: 1 out]
                n5375 = Equal To 0?(x=w3411) -> (x = 0?=w3408:bool)
                n5376 = case shown="Faux" w3408 {
                  frame False {
                  }
                  frame True {
                    n5377 = disable-structure shown="Enabled" {
                      frame Disabled {
                        n5378 = call "DCON-Read.vi"("VRN in"="HexTemp VRN") -> ("DataCluster"=→"Hexapode Temperatures":T13, "Boolean array"=→"Hexapod Alarms":bool[], "error out"=w3415:errorcluster)  [unwired: 11 in, 1 out]
                        n5379 = local write "HexapodeTempError"(w3415) -> ()
                        n5380 = Unbundle By Name(w3415) -> ("status"=w3418:bool)
                        n5381 = Not(x=w3418) -> (.not. x?=→"HexTemp COMM":bool)
                      }
                      frame Enabled {
                      }
                    }
                  }
                }
              }
              event "Setting", "Focus slew": Value Change {
                n5382 = event-data() -> ()  [unwired: 1 in, 6 out]
                n5383 = local read "Focus slew"() -> (w3467:bool)
                n5384 = local read "Setting"() -> (w3469:bool)
                n5385 = Not(x=w3467) -> (.not. x?=w3466:bool)
                n5386 = case shown="Faux" w3469 {
                  selector: w3469 -> [_ w3475]
                  tunnel: [w3470 w3475] -> w3468
                  frame False {
                    n5387 = local read "Foyer"() -> (w3473:dbl)
                    n5388 = local read "Foyer Nominal"() -> (w3474:dbl)
                    n5389 = Subtract(x=w3474, y=w3473) -> (x-y=w3472:dbl)
                    n5390 = Greater?(x=w3472, y=1.0) -> (0:w3470:bool)
                  }
                  frame True {
                  }
                }
                n5391 = And(x=w3466, y=w3468) -> (x .and. y?=w3465:bool)
                n5392 = case shown="Faux" w3465 {
                  frame False {
                    # "Ici, normalement, on est à la fin d'une séquence de foyer ..."
                    n5393 = local read "Foyer"() -> (w3476:dbl)
                    n5394 = Get Date/Time In Seconds() -> (seconds since 1Jan1904=w3478:timestamp)
                    n5395 = To Extended Precision Float(1:w3478) -> (0:→"last_foc_chg":ext)
                    n5396 = local write "Foyer Nominal"(w3476) -> ()
                    n5397 = local read "indic-T-struct"() -> (→"tmp.str":dbl)
                    "CheckFocus" <- TRUE
                  }
                  frame True {
                  }
                }
              }
              event "Recalculer": Value Change {
                # "Ne devrait pas être fait sur une base régulière, mais simplement quand les paramètres ont changés ...\n\nC'est ici qu'on veut cleaner les dossiers de data et construire les mosaiques d'image et de données !!!\n\nPour l'instant, tout a été arraché le temps de débuggé les Queries USNO & DSS !!!"
                n5398 = event-data() -> ()  [unwired: 1 in, 6 out]
                n5399 = case shown="Vrai" "Recalculer" {
                  selector: "Recalculer" -> [_ w3488]
                  frame False {
                  }
                  frame True {
                    n5400 = stacked-sequence {
                      seq-local: [w3495 _ _ _] -> [_ w3499 w3527 _]
                      seq-local: [w3494 _ _ _] -> [_ w3500 w3526 _]
                      tunnel: w3488 -> [_ _ _ _]
                      frame #0 {
                        w3496 = FALSE ("DSS_ready")
                        # "Époque DSS et USNO"
                        # "Ici il faudra s'assurer que l'astrométrie tourne autour du centre, mais\nutilise la position synchronisée comme valeur de référence"
                        # "Ces variables sont probablement\nmaintenant inutiles"
                        # "à remettre éventuellement ..."
                        # "Calcul les paramètres du champ ..."
                        n5401 = disable-structure shown="Disabled" {
                          frame Disabled {
                          }
                          frame Enabled {
                          }
                        }
                        n5402 = local read "Img DEC"() -> (w3491:dbl)
                        n5403 = local read "Img RA"() -> (w3490:dbl)
                        n5404 = local read "Epoch Tel"() -> (w3493:dbl)
                        n5405 = call "precess.vi"("Eq2"=2000.0, "Eq1"=w3493, "DEC 1"=w3491, "RA 1"=w3490) -> ("DEC 2"=w3495:dbl, "RA 2"=w3494:dbl)
                        n5406 = local write "USNO_ready"(FALSE) -> ()
                        n5407 = local write "Indicateur d'état"("Calcul des paramètres du champ") -> ()
                        "DSS_ready" <- w3496
                        "USNO_ready" <- w3496
                      }
                      frame #1 {
                        # "Télécharge les données USNO associées ..."
                        # "DEC centre img"
                        # "RA centre img"
                        n5408 = flat-sequence {
                          tunnel: w3500 -> [w3510]
                          tunnel: w3499 -> [w3509]
                          tunnel: [w3504] -> w3498
                          tunnel: w3498 -> [w3522]
                          frame #0 {
                            # "R1mag limite USNO"
                            n5409 = local read "Représentation"() -> (w3501:dbl)
                            n5410 = local read "path_data"() -> (w3506:path)
                            n5411 = while {
                              stop <- w3512 stop-if-true
                              n5412 = local read "BestTargetLed"() -> (w3514:bool)
                              n5413 = Wait (ms)(milliseconds to wait=u32 333) -> ()  [unwired: 1 out]
                              n5414 = Not(x=w3514) -> (.not. x?=w3513:bool)
                              n5415 = local write "BestTargetLed"(w3513) -> ()
                              n5416 = local read "USNO_ready"() -> (w3512:bool)
                            }
                            n5417 = local read "wgetexec"() -> (w3505:path)
                            n5418 = call "QueryUSNO.vi"("wget"=w3505, "Data dir Path"=w3506, "mag_limit"=12.0, "radius"=w3501, "DEC"=w3509, "RA"=w3510) -> ("Data OUT"=w3507:string[][], "No Error"=w3502:bool)  [unwired: 3 in, 1 out]
                            n5419 = case shown="Vrai" w3502 {
                              tunnel: w3507 -> [_ w3521]
                              tunnel: w3502 -> [w3516 w3518]
                              tunnel: [w3516 w3518] -> w3504
                              tunnel: [TRUE TRUE] -> w3503
                              frame False {
                              }
                              frame True {
                                # "6 = R1mag"
                                n5420 = call "Sort_USNO_data.vi"("Column Used"=6, "Data IN"=w3521) -> ("Data OUT"=→"USNO_data":string[][])  [unwired: 8 in, 1 out]
                              }
                            }
                            n5421 = local write "USNO_ready"(w3503) -> ()
                          }
                          frame #1 {
                            n5422 = local write "USNO_ready"(w3522) -> ()
                            n5423 = local write "BestTargetLed"(w3522) -> ()
                          }
                        }
                      }
                      frame #2 {
                        # "Pour que l'image disparaisse quand\non coche ou décoche l'option du menu"
                        # "Get the dss image ...\nÉventuellement va vérifier l'existence et créer les mosaïques\nPour l'instant, on ne le permet qu'avec le bouton \"GetDSS\""
                        n5424 = local read "Img RA"() -> (w3537:dbl)
                        n5425 = local read "imageDSS"() -> (w3524:bool)
                        n5426 = local read "Img DEC"() -> (w3528:dbl)
                        n5427 = Subtract(x=w3526, y=w3537) -> (x-y=w3535:dbl)
                        n5428 = Subtract(x=w3527, y=w3528) -> (x-y=w3536:dbl)
                        n5429 = Absolute Value(x=w3535) -> (abs(x)=w3534:dbl)
                        n5430 = Absolute Value(x=w3536) -> (abs(x)=w3533:dbl)
                        n5431 = Greater?(x=w3534, y=1.0) -> (0:w3529:bool)
                        n5432 = Not(x=w3524) -> (.not. x?=w3523:bool)
                        n5433 = Greater?(x=w3533, y=1.0) -> (0:w3530:bool)
                        n5434 = Compound Arithmetic op=OR(w3529, w3530, w3523) -> (w3525:bool)
                        n5435 = case shown="Vrai" w3525 {
                          tunnel: w3526 -> [_ w3540]
                          tunnel: w3527 -> [_ w3541]
                          frame False {
                            n5436 = local read "imageDSS"() -> (w3538:bool)
                            n5437 = local write "DSS_ready"(w3538) -> ()
                          }
                          frame True {
                            n5438 = local read "imageDSS"() -> (w3539:bool)
                            n5439 = case shown="Vrai" w3539 {
                              tunnel: w3541 -> [_ w3546]
                              tunnel: w3540 -> [_ w3545]
                              frame False {
                                n5440 = property on="TableXYPos" class="GraphXY (strict)"("PlotImages.Back"=picture data[5B] ("Images")) -> ()  [unwired: 2 in, 2 out]
                              }
                              frame True {
                                n5441 = flat-sequence {
                                tunnel: w3545 -> [w3556]
                                tunnel: w3546 -> [w3557]
                                tunnel: [w3557] -> w3544
                                tunnel: [w3556] -> w3543
                                tunnel: w3544 -> [w3566]
                                tunnel: w3543 -> [w3565]
                                frame #0 {
                                w3547 = u16 1 items=["Region d'intérêt", "Prévisualisation"] ("ImageUsage")
                                w3552 = 0
                                n5442 = Initialize Array(sgl 0.0, w3552, w3552) -> (w3551:sgl[][])
                                n5443 = local write "ImgData"(w3551) -> ()
                                n5444 = local write "SubIMG4DSS?"(TRUE ("SubIMG4DSS?")) -> ()
                                n5445 = local write "ImgAstrom"(T4 {"NAXIS"=[], "CD"=[], "CDELT"=[], "CRPIX"=[], "CTYPE"=[], "CRVAL"=[], "LONGPOLE"=180.0, "LATPOLE"=90.0, "PV2"=[]} ("ImgAstrom")) -> ()
                                n5446 = call "Draw_crosshair.vi"("Image IN"=w3551, "White Value"=sgl 255.0) -> ("Image OUT"=w3550:sgl[][])  [unwired: 13 in]
                                n5447 = property on="TableXYPos" class="GraphXY (strict)"("PlotImages.Back"=picture data[5B] ("Images")) -> ()  [unwired: 2 in, 2 out]
                                n5448 = local write "subimg"(w3550) -> ()
                                n5449 = local write "ImageUsage"(w3547) -> ()
                                }
                                frame #1 {
                                # "Ici, le code devrait vérifier l'existence des images sur le disque ..."
                                n5450 = local read "Représentation"() -> (w3560:dbl)
                                n5451 = local read "path_dss"() -> (w3563:path)
                                n5452 = local read "wgetexec"() -> (w3562:path)
                                n5453 = Add(x=4.0, y=w3560) -> (x+y=w3558:dbl)
                                n5454 = call "Query_Vizier.vi"("Folder"=w3563, "wget"=w3562, "Width"=w3558, "Height"=w3558, "DEC"=w3566, "RA"=w3565) -> ("error?"=w3561:bool, "Path2Image"=w3569:path)  [unwired: 4 in]
                                "Path2Image" <- w3569
                                n5455 = case shown="Faux" w3561 {
                                tunnel: w3565 -> [w3574 _]
                                tunnel: w3566 -> [w3573 _]
                                tunnel: w3569 -> [w3576 _]
                                tunnel: [w3574 -inf ("RA OUT")] -> w3568
                                tunnel: [w3573 -inf ("RA OUT")] -> w3567
                                tunnel: [TRUE FALSE] -> w3564
                                frame False {
                                # "ImgData et ImgAstrom\nsont lié à plus grand que le\nchamp affiché."
                                n5456 = property on="TableXYPos" class="GraphXY (strict)"() -> ("Height"=w3582:u32, "Width"=w3581:u32)  [unwired: 2 in, 2 out]
                                n5457 = local read "FieldAstrom"() -> (w3572:T4)
                                n5458 = property on="TableXYPos" class="GraphXY (strict)"() -> ("XScale.Range"=w3578:T26, "YScale.Range"=w3577:T26)  [unwired: 2 in, 2 out]
                                n5459 = To Long Integer(number=w3582) -> (32bit integer=w3580:i32)
                                n5460 = To Long Integer(number=w3581) -> (32bit integer=w3579:i32)
                                n5461 = call "Draw_graph_background.vi"("Y Scale.Range"=w3577, "ImgRA"=w3574, "X Scale.Range"=w3578, "ImgDEC"=w3573, "Field Astrometry"=w3572, "New Width"=w3579, "New Height"=w3580, "path"=w3576) -> ("ImgData"=→"ImgData":sgl[][], "Astrometry"=→"ImgAstrom":T4, "Images"=w3571:picture)  [unwired: 1 out]
                                n5462 = property on="TableXYPos" class="GraphXY (strict)"("PlotImages.Back"=w3571) -> ()  [unwired: 2 in, 2 out]
                                }
                                frame True {
                                }
                                }
                                "Img RA" <- w3568
                                "Img DEC" <- w3567
                                n5463 = local write "DSS_ready"(w3564) -> ()
                                }
                                }
                              }
                            }
                          }
                        }
                      }
                      frame #3 {
                        # "Retrace l'image de la caméra de référence ..."
                        n5464 = local write "Recalculer"(FALSE ("Recalculer")) -> ()
                      }
                    }
                  }
                }
                n5465 = while {
                  tunnel: [FALSE] -> w3481
                  stop <- w3487 continue-if-true
                  n5466 = local read "Downloading ..."() -> (w3485:bool)
                  n5467 = Not(x=w3485) -> (.not. x?=→"Downloading ...":bool)
                  n5468 = Wait (ms)(milliseconds to wait=u32 333) -> ()  [unwired: 1 out]
                  n5469 = local read "Recalculer"() -> (w3487:bool)
                }
                n5470 = local write "Downloading ..."(w3481) -> ()
              }
              event "Slewing": Value Change {
                n5471 = event-data() -> ("NewVal"=w3588:bool)  [unwired: 1 in, 5 out]
                n5472 = case shown="Faux" w3588 {
                  frame False {
                    w3590 = FALSE ("Blinking")
                    w3591 = 0
                    # "Fin d'un déplacement ..."
                    # "Activer les boutons"
                    n5473 = property on="Zénith" class="Bool (strict)"("Blinking"=w3590) -> ()  [unwired: 2 in, 2 out]
                    n5474 = property on="Range" class="Bool (strict)"("Blinking"=w3590) -> ()  [unwired: 2 in, 2 out]
                    n5475 = property on="Écran" class="Bool (strict)"("Blinking"=w3590) -> ()  [unwired: 2 in, 2 out]
                    n5476 = property on="GO" class="Bool (strict)"("Disabled"=w3591) -> ()  [unwired: 2 in, 2 out]
                    n5477 = property on="Synctel" class="Bool (strict)"("Disabled"=w3591) -> ()  [unwired: 2 in, 2 out]
                    n5478 = property on="ModifRotation" class="Bool (strict)"("Disabled"=w3591) -> ()  [unwired: 2 in, 2 out]
                    n5479 = property on="Offset OK" class="Bool (strict)"("Disabled"=w3591) -> ()  [unwired: 2 in, 2 out]
                    n5480 = property on="ModifFoyer" class="Bool (strict)"("Disabled"=w3591) -> ()  [unwired: 2 in, 2 out]
                    n5481 = property on="Écran" class="Bool (strict)"("Disabled"=w3591) -> ()  [unwired: 2 in, 2 out]
                    n5482 = property on="Zénith" class="Bool (strict)"("Disabled"=w3591) -> ()  [unwired: 2 in, 2 out]
                    n5483 = property on="Range" class="Bool (strict)"("Disabled"=w3591) -> ()  [unwired: 2 in, 2 out]
                    n5484 = property on="ModCoor" class="Bool (strict)"("Disabled"=w3591) -> ()  [unwired: 2 in, 2 out]
                    n5485 = property on="ModifDome" class="Bool (strict)"("Disabled"=w3591) -> ()  [unwired: 2 in, 2 out]
                    n5486 = local read "Déplacement usager"() -> (w3589:bool)
                    n5487 = case shown="Vrai" w3589 {
                      frame False {
                        w3592 = FALSE ("Déplacement usager")
                        n5488 = local write "Déplacement usager"(w3592) -> ()
                        n5489 = local write "From library"(w3592) -> ()
                      }
                      frame True {
                        w3601 = "\t"
                        w3607 = "_"
                        w3613 = TRUE ("replace all? (F)")
                        w3614 = " "
                        w3615 = "0"
                        w3618 = i16 2 ("width (-)")
                        w3619 = i16 0 ("width (-)")
                        # "Devrait aussi être mis dans un log pour pouvoir y revenir plus tard ..."
                        # "Enregistre la nouvelle position du télescope"
                        n5490 = local write "Déplacement usager"(FALSE ("Déplacement usager")) -> ()
                        n5491 = local read "Epoch Tel"() -> (w3623:dbl)
                        n5492 = local read "DEC Tel"() -> (w3621:dbl)
                        n5493 = local read "RA Tel"() -> (w3622:dbl)
                        n5494 = call "time-sec-to-time-str-DEC.vi"("Numeric"=w3622) -> ("formatted-str"=w3604:string)
                        n5495 = call "time-sec-to-time-str-DEC.vi"("Numeric"=w3621) -> ("formatted-str"=w3603:string)
                        n5496 = Number To Fractional String(number=w3623, width (-)=i16 4, precision (6)=i16 2) -> (F-format string=w3602:string)  [unwired: 1 in]
                        n5497 = Get Date/Time String() -> (time string=w3605:string)  [unwired: 3 in, 1 out]
                        n5498 = local read "From library"() -> (w3627:bool)
                        n5499 = Concatenate Strings(w3605, w3601, w3604, w3601, w3603, w3601, w3602, "\r\n") -> (w3593:string)
                        n5500 = call "GetUTC.vi"() -> ("Day"=w3597:dbl, "Month"=w3598:dbl, "Year"=w3599:dbl)  [unwired: 6 out]
                        n5501 = case shown="Vrai" w3627 {
                          tunnel: [FALSE FALSE] -> w3626
                          tunnel: w3604 -> [w3632 w3639]
                          tunnel: w3603 -> [w3631 w3640]
                          tunnel: w3602 -> [w3630 w3641]
                          tunnel: w3605 -> [w3629 w3638]
